vi "array_of_azimuts.vi"(10 "Cluster in":T1, 11 "pieceOfWorld":T2[][](array[typedef])) -> (3 "Cluster out":T1)   [LabVIEW 2015, in "PolyVIEW.lvclass"]
uses:
  PolyVIEW.lvclass
  actors/world/typedefs/worldCell_cluster.ctl
  actors/world/typedefs/markValue_cluster.ctl
  actors/world/typedefs/markValue.ctl
  actors/world/typedefs/markVolume.ctl
  actors/world/typedefs/amountOfFood.ctl
  actors/world/typedefs/anthillType_enum.ctl
  Admin memo.ctl
  actors/world/world.lvlib
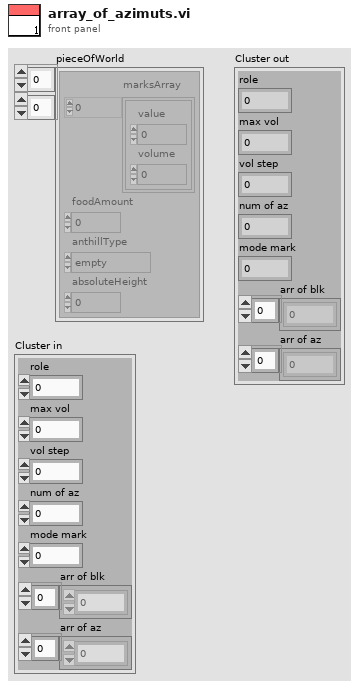
[diagram p1: front panel]
types:
  T1 = typedef "PolyVIEW.lvclass/Admin memo.ctl" = cluster{"role":i32, "max vol":i32, "vol step":i32, "num of az":i32, "mode mark":i32, "arr of blk":i32[], "arr of az":i32[]}
  T2 = typedef "world.lvlib/worldCell_cluster.ctl" = cluster{"marksArray":T3[], "foodAmount":T6, "anthillType":T7, "absoluteHeight":u8}
  T3 = typedef "world.lvlib/markValue_cluster.ctl" = cluster{"value":T4, "volume":T5}
  T4 = typedef "world.lvlib/markValue.ctl" = u8
  T5 = typedef "world.lvlib/markVolume.ctl" = u16
  T6 = typedef "world.lvlib/amountOfFood.ctl" = i32
  T7 = typedef "world.lvlib/anthillType_enum.ctl" = enum16{"empty", "own", "rival"}
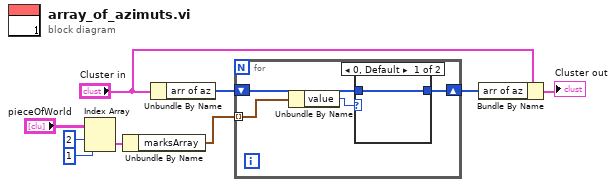
[diagram p0: block diagram]
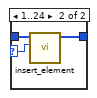
[diagram p2: hidden frame]
diagram:
  n1 = Index Array(array="pieceOfWorld", index (row)=2, index (col)=1 ("disabled index (col)")) -> (element=w6:T2)
  n2 = Unbundle By Name(w6) -> ("marksArray"=w7:T3[])
  n3 = Unbundle By Name("Cluster in") -> ("arr of az"=w8:i32[])
  n4 = for {
    tunnel: w7 -> [w11] mode=indexing
    shift-right: [w12] -> w9
    shift-left: w8 -> [w13]
    n5 = Unbundle By Name(w11) -> ("value"=w10:T4)
    n6 = case shown="0, Default" w10 {
      selector: w10 -> [_ w15]
      tunnel: w13 -> [w14 w17]
      tunnel: [w14 w16] -> w12
      frame 0, Default {
      }
      frame 1..24 {
        n7 = call "insert_element.vi"("element"=w15, "array in"=w17) -> ("array out"=w16:i32[])  [unwired: 9 in]
      }
    }
  }
  n8 = Bundle By Name(cluster="Cluster in", "arr of az"=w9) -> (→"Cluster out":T1)
